vi "Write_Table_To_XL_OPEN.vi"(0 "Table":string[][](table)=[["510,000000000000", "1,000000000000", "1000000,000000000000", "100000,000000000000", "-18,607472685587", "-56,309709692621", "-72,645996842461", "-19,372830852352", "0,080012670618", "-0,000045516539", "1,555401708353", "0,014865172083", "-0,299720385656", "0,000006753800", "-0,000313765807", "1,114555386279", "1,043587015218", "-0,299719185267", "0,000119711658", "0,015571898704", "2,072394143790", "0,000000000000", "-0,005061278170", "0,000000000000", "0,015309123648", "1,631256718730", "2,000000000000", "-0,005060079859", "0,010000000000", "0,000000500000", "0,000000200000", "0,000000500000", "0,000000200000", "0,000001000000", "0,000001000000", "0,000001000000", "0,000001000000", "0,000001000000", "0,000001000000", "0,000001000000", "0,000001000000", "0,000050000000", "0,000030000000", "0,000050000000", "0,000030000000", "0,000000500000", "0,000000200000", "0,000000500000", "0,000000200000", "0,000000002000", "0,000000000000", "-0,000045516539", "0,015571898704"]], 1 "Excel._Workbook":refnum<k7>, 5 "SheetName":string, 11 "error in (no error)":errorcluster, 12 "Page index":i32=1) -> (15 "error out":errorcluster)   [LabVIEW 2014]
doc: "This VI demonstrates the basic idea of using the OLE Automation VIs by writing a Table into an Excel WorkSheet."
panel:
  # "This VI demostrates the basic steps needed to enter the values in a table into a spreadsheet and then save it to a file."
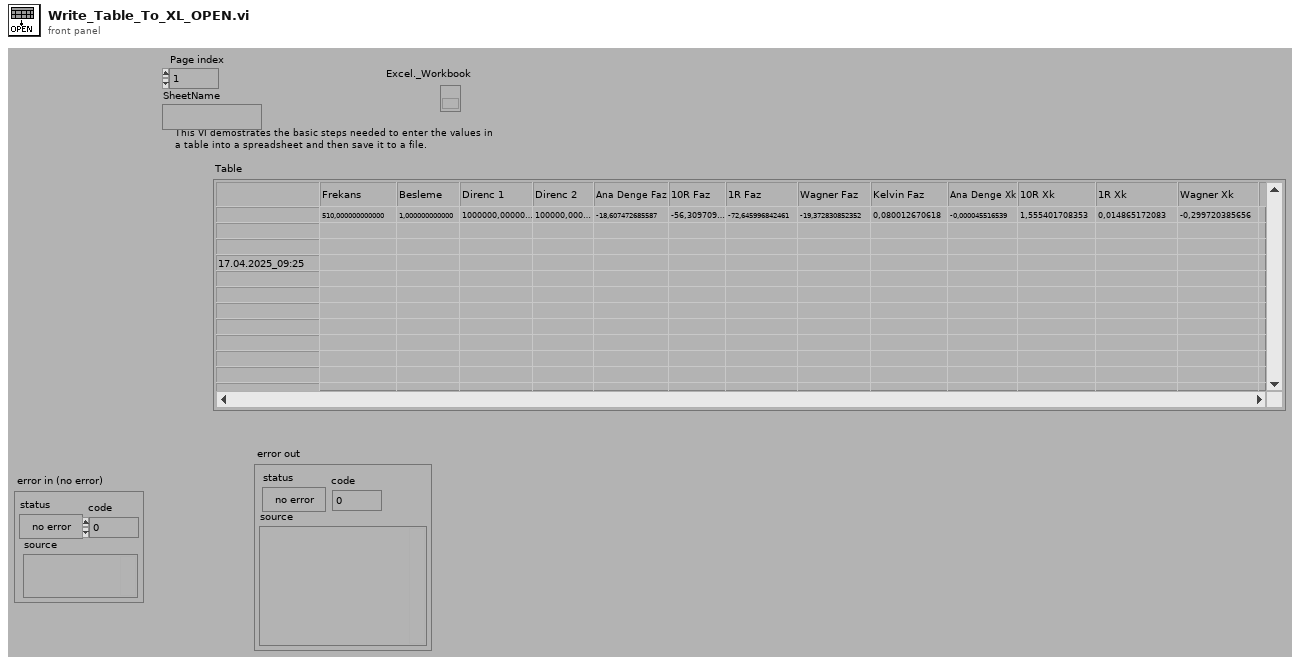
[diagram p1: front panel]
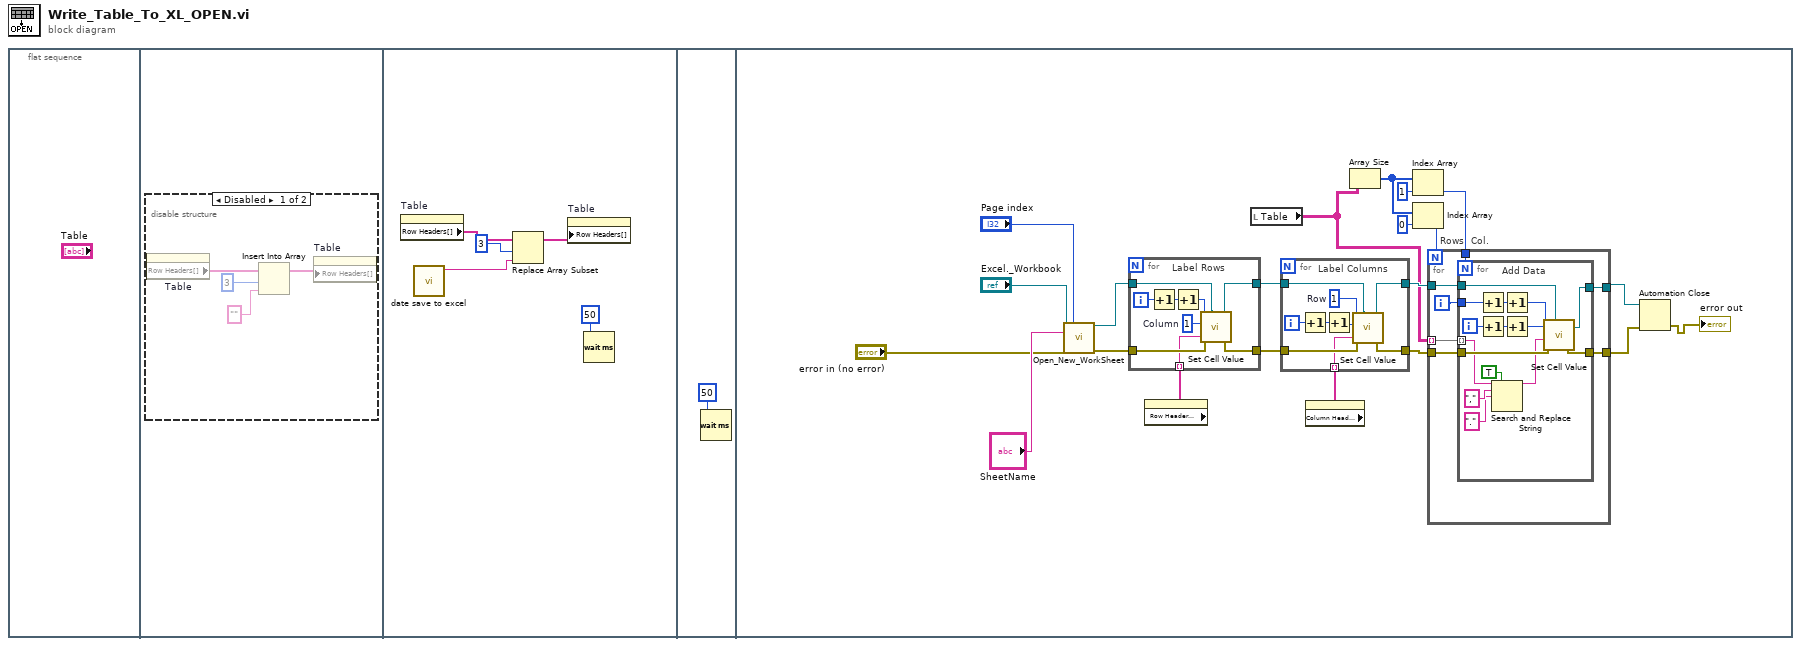
[diagram p0: block diagram]
diagram:
  n1 = flat-sequence {
    frame #0 {
    }
    frame #1 {
      n2 = disable-structure shown="Disabled" {
        frame Disabled {
          n3 = property on="Table" class="Tbl (strict)"() -> ("Row Headers[]"=w2:string[])  [unwired: 2 in, 2 out]
          n4 = Insert Into Array(array=w2, index=3, new element="" ("new element/subarray")) -> (w4:string[])
          n5 = property on="Table" class="Tbl (strict)"("Row Headers[]"=w4) -> ()  [unwired: 2 in, 2 out]
        }
        frame Enabled {
        }
      }
    }
    frame #2 {
      n6 = property on="Table" class="Tbl (strict)"() -> ("Row Headers[]"=w9:string[])  [unwired: 2 in, 2 out]
      n7 = call "date save to excel.vi"() -> ("concatenated string"=w7:string)  [unwired: 11 in]
      n8 = Replace Array Subset(array=w9, new element=w7, index=3) -> (w6:string[])
      n9 = property on="Table" class="Tbl (strict)"("Row Headers[]"=w6) -> ()  [unwired: 2 in, 2 out]
      n10 = Wait (ms)(milliseconds to wait=u32 50) -> ()  [unwired: 1 out]
    }
    frame #3 {
      n11 = Wait (ms)(milliseconds to wait=u32 50) -> ()  [unwired: 1 out]
    }
    frame #4 {
      # "Col."
      # "Rows"
      n12 = call "Open_New_WorkSheet.vi"("Excel._Workbook"="Excel._Workbook", "Page index"="Page index", "SheetName"="SheetName", "error in (no error)"="error in (no error)") -> ("Excel._Worksheet"=w16:refnum<k7>, "error out"=w17:errorcluster)  [unwired: 10 out]
      n13 = property on="Property Node" class="Tbl (strict)"() -> ("Row Header Strings[]"=w28:string[])  [unwired: 2 in, 2 out]
      n14 = for {
        tunnel: w16 -> [w67]
        tunnel: w17 -> [w66]
        tunnel: [w65] -> w25
        tunnel: [w64] -> w26
        tunnel: w28 -> [w63] mode=indexing
        i -> [w71]
        w69 = 1  # Column
        # "Label Rows"
        n15 = Increment(x=w71) -> (x+1=w70:i32)
        n16 = Increment(x=w70) -> (x+1=w68:i32)
        n17 = call "Set Cell Value.vi"("Row"=w68, "Col"=w69, "Value"=w63, "error in (no error)"=w66, "Excel._Worksheet"=w67) -> ("Excel._Worksheet"=w64:refnum<k7>, "error out"=w65:errorcluster)
      }
      n18 = local read "Table"() -> (w11:string[][])
      n19 = property on="Table" class="Tbl (strict)"() -> ("Column Header Strings[]"=w27:string[])  [unwired: 2 in, 2 out]
      n20 = for {
        tunnel: w26 -> [w38]
        tunnel: w25 -> [w37]
        tunnel: [w36] -> w23
        tunnel: [w35] -> w24
        tunnel: w27 -> [w32] mode=indexing
        i -> [w40]
        w33 = 1  # Row
        # "Label Columns"
        n21 = Increment(x=w40) -> (x+1=w39:i32)
        n22 = Increment(x=w39) -> (x+1=w34:i32)
        n23 = call "Set Cell Value.vi"("Row"=w33, "Col"=w34, "Value"=w32, "error in (no error)"=w37, "Excel._Worksheet"=w38) -> ("Excel._Worksheet"=w35:refnum<k7>, "error out"=w36:errorcluster)
      }
      n24 = Array Size(array=w11) -> (size(s)=w31:i32[])
      n25 = Index Array(array=w31, index=1) -> (element=w22:i32)
      n26 = Index Array(array=w31, index=0) -> (element=w21:i32)
      n27 = for {
        N: w21 -> [_]
        tunnel: w24 -> [w47]
        tunnel: w23 -> [w44]
        tunnel: [w46] -> w20
        tunnel: w11 -> [w43] mode=indexing
        tunnel: w22 -> [w42]
        tunnel: [w41] -> w19
        i -> [w45]
        n28 = for {
          N: w42 -> [_]
          tunnel: w47 -> [w57]
          tunnel: w44 -> [w56]
          tunnel: [w55] -> w46
          tunnel: w45 -> [w54]
          tunnel: w43 -> [w52] mode=indexing
          tunnel: [w53] -> w41
          i -> [w62]
          # "Add Data"
          n29 = Increment(x=w54) -> (x+1=w61:i32)
          n30 = Increment(x=w62) -> (x+1=w59:i32)
          n31 = Search and Replace String(replace all?=TRUE ("replace all? (F)"), input string=w52, search string=",", replace string="." ("replace string (\"\")")) -> (result string=w51:string)  [unwired: 1 in, 6 out]
          n32 = Increment(x=w61) -> (x+1=w60:i32)
          n33 = Increment(x=w59) -> (x+1=w58:i32)
          n34 = call "Set Cell Value.vi"("Row"=w60, "Col"=w58, "Value"=w51, "error in (no error)"=w56, "Excel._Worksheet"=w57) -> ("Excel._Worksheet"=w53:refnum<k7>, "error out"=w55:errorcluster)
        }
      }
      n35 = Automation Close(3:w20, 5:w19) -> (0:→"error out":errorcluster)
    }
  }
